vi "读取数据库.vi"(7 "condition":string, 8 "error in (no error)":errorcluster caption="错误输入（无错误）", 9 "database":string="database1.mdb", 10 "显示项":string[](array[string]), 11 "组合框":string(combo)) -> (0 "error out":errorcluster caption="错误输出", 1 "columns":string[](array[string]), 2 "data":variant[][](array[variant]), 3 "表格":string[][](table))   [LabVIEW 2016, in "数据查询.lvlib"]
uses:
  <vilib>/Utility/sysdir.llb/System Directory Type.ctl
  <vilib>/addons/database/Connection.llb/DB Tools Open Connec (String).vi
  <vilib>/addons/database/_DB Variant To Data/Database Variant To Data.xnode
  <vilib>/addons/database/NI_Database_API.lvlib
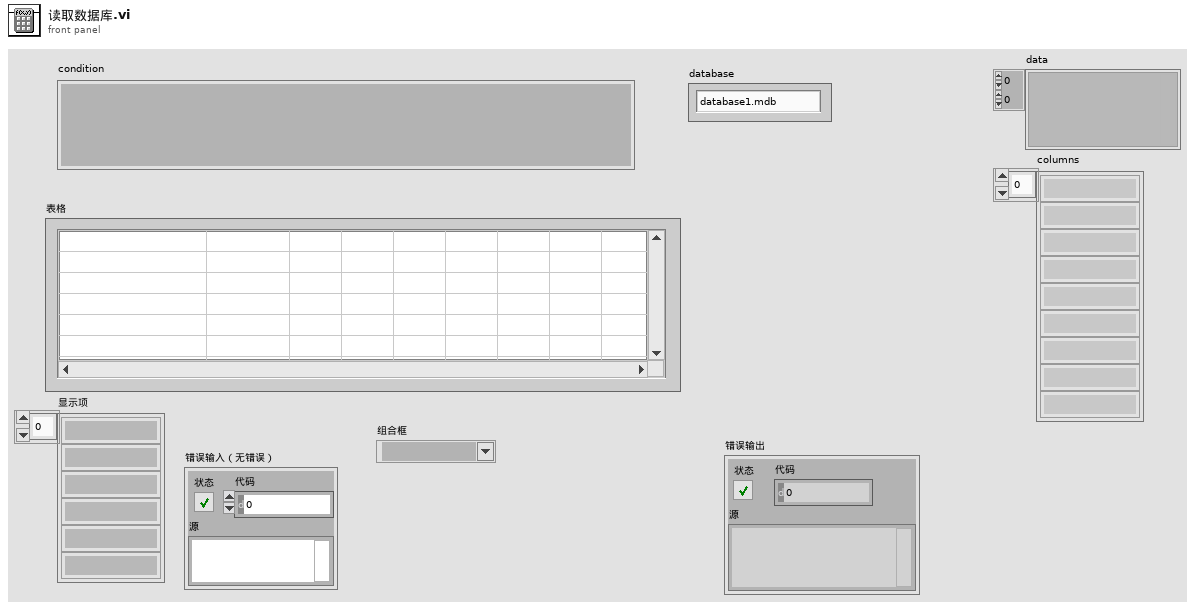
[diagram p1: front panel]
types:
  T1 = typedef "System Directory Type.ctl" = i32
  T2 = typedef "NI_Database_API.lvlib/Conn ObjectReference.ctl" = refnum<k1>
  T3 = typedef "NI_Database_API.lvlib/DB Tools DataTypes.ctl" = enum16{"String", "Long (I32)", "Single (SGL)", "Double (DBL)", "Date/Time", "Binary"}
  T4 = cluster{"name":string, "database data type":T3, "defined size":i32}[]
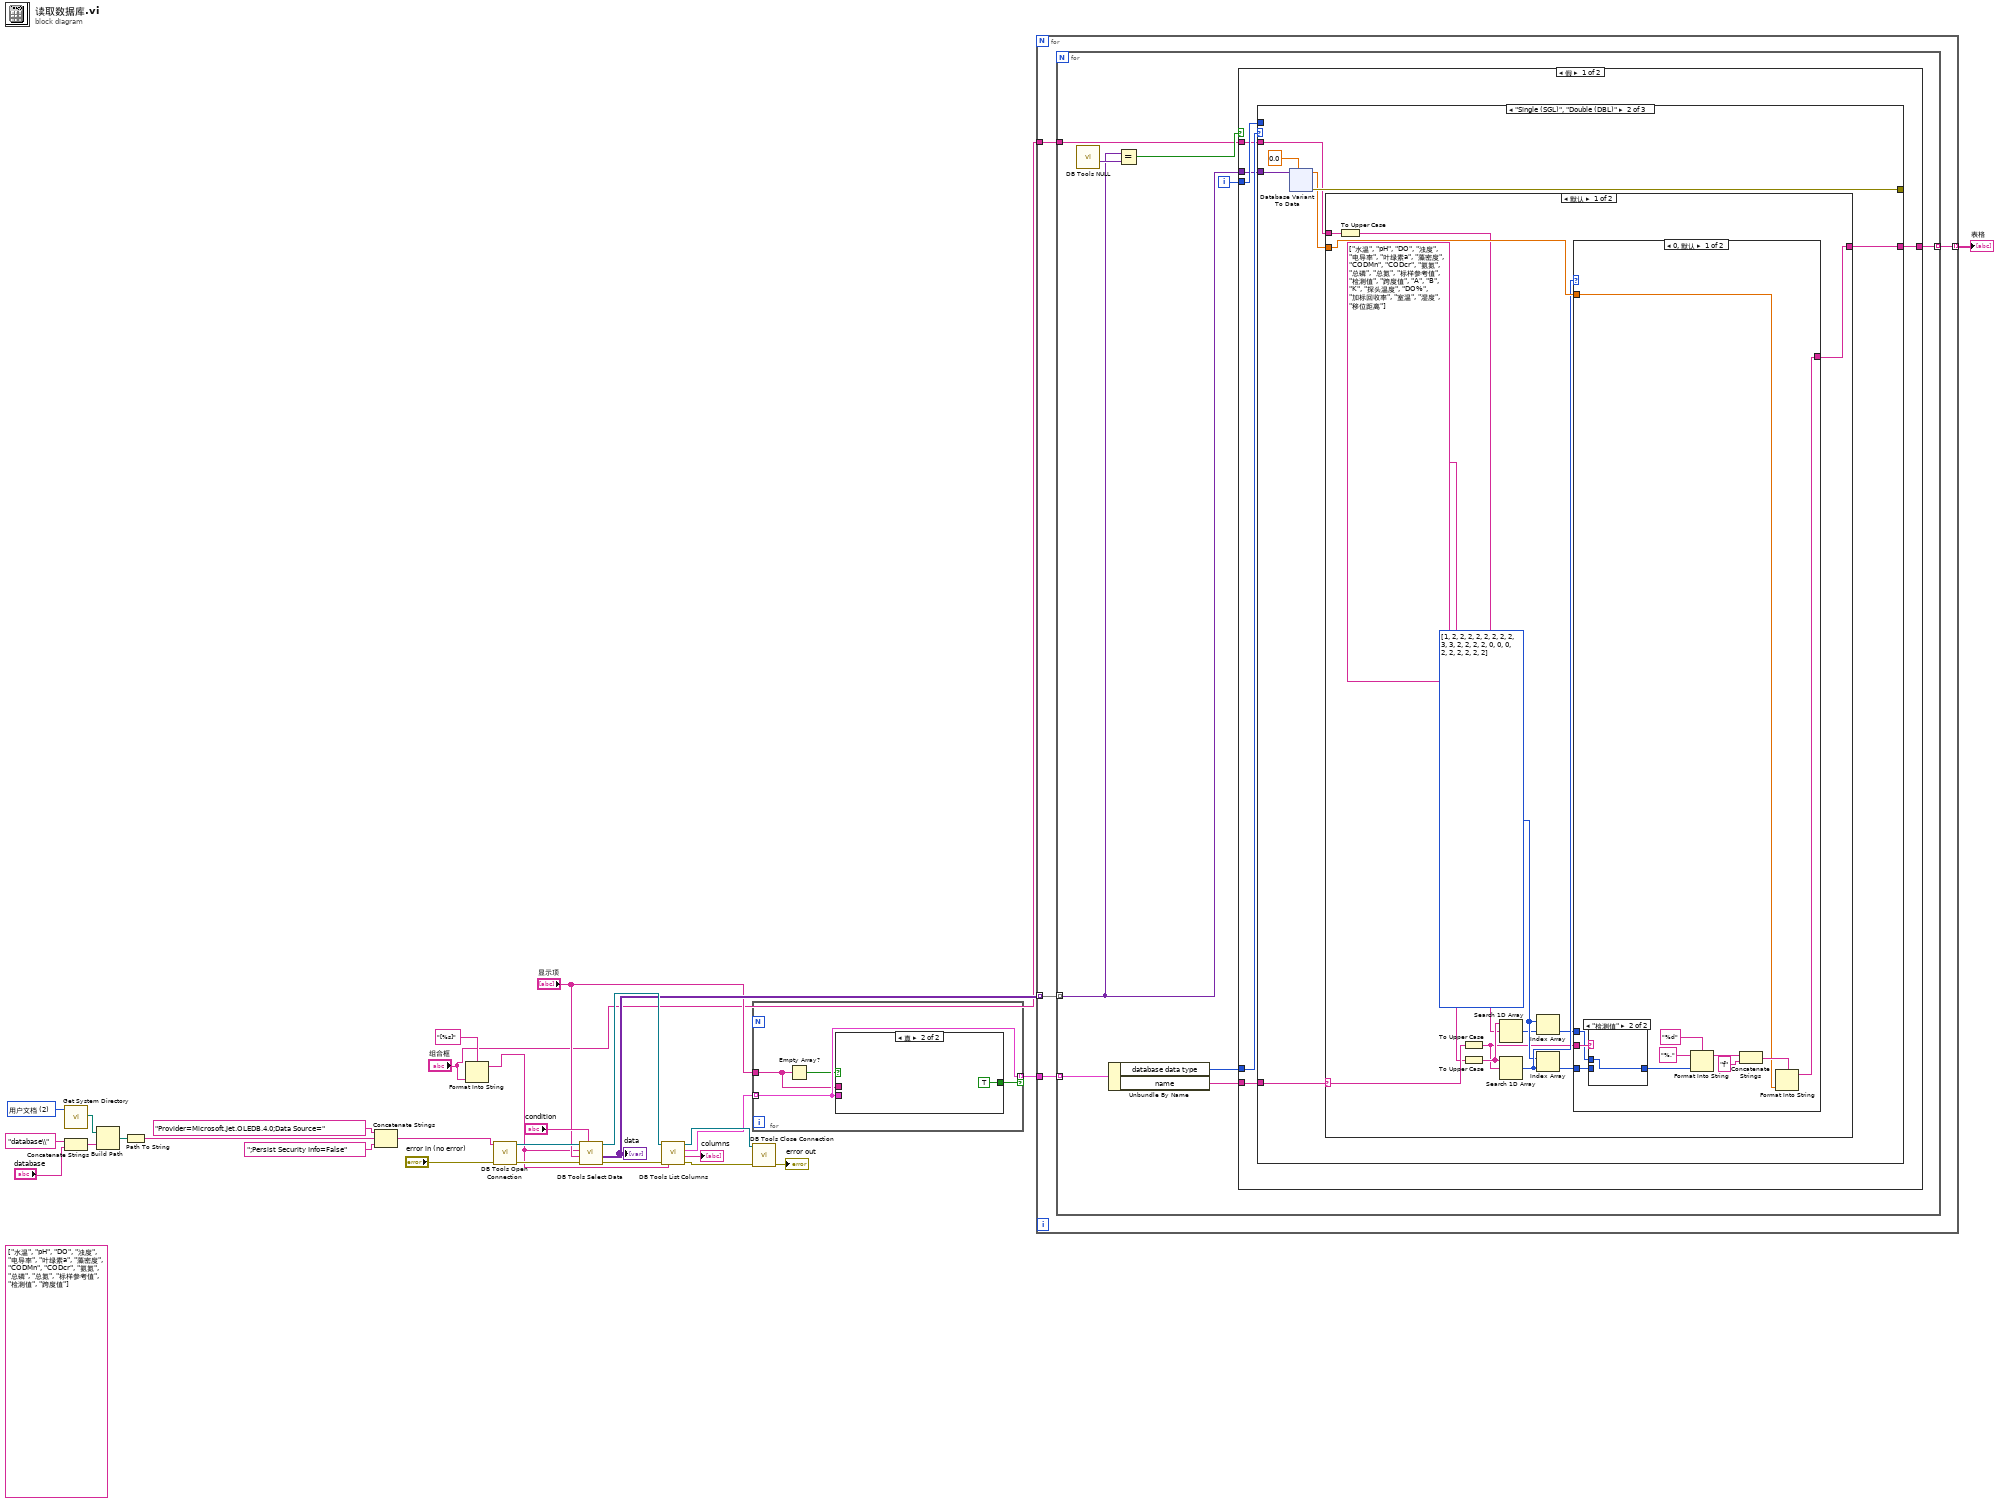
[diagram p0: block diagram]
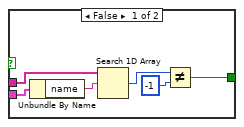
[diagram p2: hidden frame]
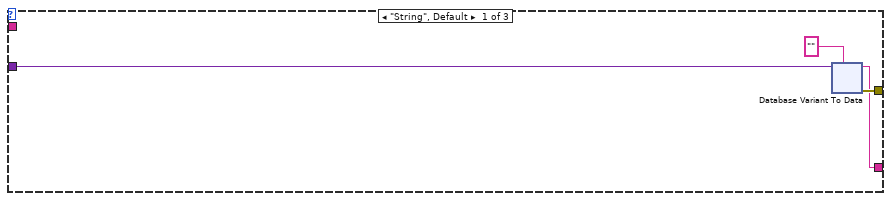
[diagram p3: hidden frame]
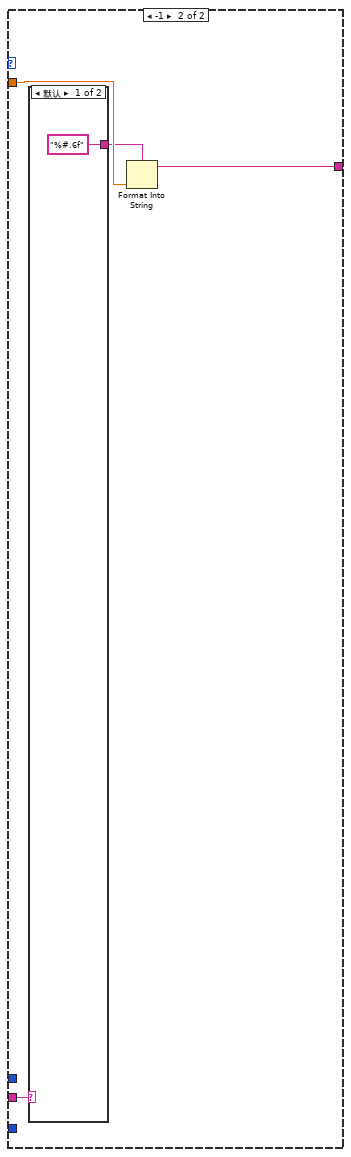
[diagram p5: hidden frame]
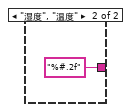
[diagram p6: hidden frame]
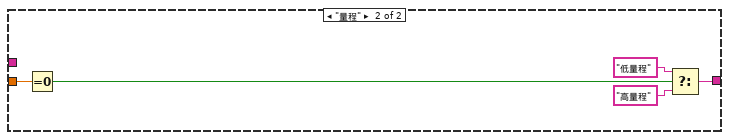
[diagram p7: hidden frame]
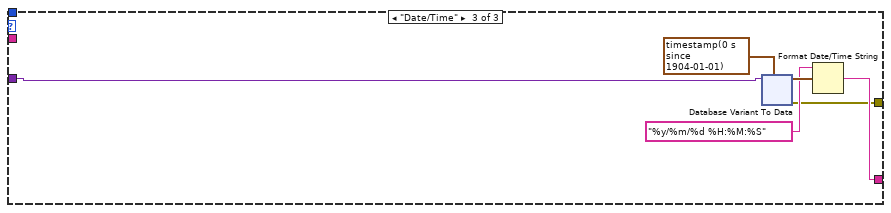
[diagram p8: hidden frame]
diagram:
  (unwired) string[] ["水温", "pH", "DO", "浊度", "电导率", "叶绿素a", "藻密度", "CODMn", "CODcr", "氨氮", "总磷", "总氮", "标样参考值", "检测值", "跨度值"]
  w15 = T1 2 items=["用户目录"=0, "用户桌面"=1, "用户文档"=2, "用户应用程序数据"=3, "用户设置"=4, "用户临时目录"=5, "公共文档"=6, "公共应用程序数据"=7, "公共设置"=8, "公共缓存"=13, "系统核心库"=9, "系统安装库"=10, "应用程序文件"=11, "启动盘根目录"=12] ("system directory type")
  n1 = call <vilib>:"Get System Directory.vi"("system directory type"=w15) -> ("system directory"=w14:path)  [unwired: 10 in]
  n2 = Concatenate Strings("database\\" ("名称或相对路径"), "database") -> (w11:string)
  n3 = Build Path(base path=w14, name or relative path=w11) -> (appended path=w16:path)
  n4 = Path To String(path=w16) -> (string=w17:string)
  n5 = Concatenate Strings("Provider=Microsoft.Jet.OLEDB.4.0;Data Source=", w17, ";Persist Security Info=False") -> (w13:string)
  n6 = Format Into String(format string="[%s]" ("格式字符串"), "组合框") -> (resulting string=w3:string)  [unwired: 2 in, 1 out]
  n7 = call-poly <vilib>:"DB Tools Open Connection.vi"("error in (no error)"="error in (no error)", "connection information"=w13) -> ("error out"=w27:errorcluster, "connection reference"=w28:T2)  [unwired: 6 in]
  n8 = call <vilib>:"DB Tools Select Data.vi"("condition"="condition", "error in (no error)"=w27, "columns"="显示项", "table"=w3, "connection reference"=w28) -> ("error out"=w26:errorcluster, "data"=w9:variant[][], "connection reference out"=w23:T2)  [unwired: 1 in]
  "data" <- w9
  n9 = call <vilib>:"DB Tools List Columns.vi"("error in (no error)"=w26, "table"=w3, "connection reference"=w23) -> ("error out"=w20:errorcluster, "columns"=→"columns":string[], "column information"=w5:T4, "connection reference out"=w21:T2)  [unwired: 1 in]
  n10 = for {
    tunnel: w5 -> [w31] mode=indexing
    tunnel: "显示项" -> [w30]
    tunnel: [w31] -> w4 mode=indexing if=w32
    n11 = Empty Array?(array=w30) -> (empty?=w29:bool)
    n12 = case shown="真" w29 {
      tunnel: [w35 TRUE] -> w32
      tunnel: w31 -> [w34 _]
      tunnel: w30 -> [w33 _]
      frame False {
        n13 = Unbundle By Name(w34) -> ("name"=w36:string)
        n14 = Search 1D Array(1D array=w33, element=w36) -> (index of element=w38:i32)  [unwired: 1 in]
        n15 = Not Equal?(x=w38, y=-1) -> (x != y?=w35:bool)
      }
      frame True {
      }
    }
  }
  n16 = call <vilib>:"DB Tools Close Connection.vi"("error in (no error)"=w20, "connection reference"=w21) -> ("error out"=→"error out":errorcluster)  [unwired: 5 in]
  n17 = for {
    tunnel: w9 -> [w43] mode=indexing
    tunnel: w4 -> [w42]
    tunnel: [w41] -> w8 mode=indexing
    tunnel: "组合框" -> [w40]
    n18 = for {
      tunnel: w43 -> [w48] mode=indexing
      tunnel: w42 -> [w52] mode=indexing
      tunnel: [w50] -> w41 mode=indexing
      tunnel: w40 -> [w46]
      i -> [w51]
      n19 = call <vilib>:"DB Tools NULL.vi"() -> ("NULL"=w49:variant)  [unwired: 10 in, 1 out]
      n20 = Unbundle By Name(w52) -> ("database data type"=w45:T3, "name"=w44:string)
      n21 = Equal?(x=w48, y=w49) -> (x = y?=w47:bool)
      n22 = case shown="假" w47 {
        tunnel: w45 -> [w58 _]
        tunnel: w51 -> [w57 _]
        tunnel: [w56 _] -> w50
        tunnel: w44 -> [w55 _]
        tunnel: w48 -> [w54 _]
        tunnel: w46 -> [w53 _]
        frame False {
          n23 = case shown="\"Single (SGL)\", \"Double (DBL)\"" w58 {
            tunnel: w54 -> [w62 w99 w176]
            tunnel: [w59 w100 w172] -> w56
            tunnel: w57 -> [_ _ _]
            tunnel: [w60 w101 w171] -> _
            tunnel: w55 -> [_ w98 _]
            tunnel: w53 -> [_ w95 _]
            frame "String", Default {
              n24 = xnode "Database Variant To Data"("database variant"=w62, "type"="") -> ("data"=w59:string, "error out"=w60:errorcluster)  [unwired: 1 in]
            }
            frame "Single (SGL)", "Double (DBL)" {
              n25 = xnode "Database Variant To Data"("database variant"=w99, "type"=0.0) -> ("data"=w96:dbl, "error out"=w101:errorcluster)  [unwired: 1 in]
              n26 = case shown="默认" w98 {
                selector: w98 -> [w112 _]
                tunnel: w96 -> [w114 w138]
                tunnel: [w113 w134] -> w100
                tunnel: w95 -> [w110 _]
                frame Default {
                  w109 = i32[] [1, 2, 2, 2, 2, 2, 2, 2, 2, 3, 3, 2, 2, 2, 2, 0, 0, 0, 2, 2, 2, 2, 2, 2]
                  n27 = To Upper Case(1:w110) -> (0:w103:string)
                  n28 = To Upper Case(1:w112) -> (0:w102:string)
                  n29 = To Upper Case(1:string[] ["水温", "pH", "DO", "浊度", "电导率", "叶绿素a", "藻密度", "CODMn", "CODcr", "氨氮", "总磷", "总氮", "标样参考值", "检测值", "跨度值", "A", "B", "K", "探头温度", "DO%", "加标回收率", "室温", "湿度", "移位距离"]) -> (0:w104:string[])
                  n30 = Search 1D Array(1D array=w104, element=w103) -> (index of element=w108:i32)  [unwired: 1 in]
                  n31 = Search 1D Array(1D array=w104, element=w102) -> (index of element=w111:i32)  [unwired: 1 in]
                  n32 = Index Array(array=w109, index=w108) -> (element=w107:i32)
                  n33 = Index Array(array=w109, index=w111) -> (element=w106:i32)
                  n34 = case shown="0, 默认" w111 {
                    tunnel: w114 -> [w119 w131]
                    tunnel: [w117 w130] -> w113
                    tunnel: w102 -> [w118 w128]
                    tunnel: w107 -> [w116 _]
                    tunnel: w106 -> [w115 _]
                    frame 0, Default {
                      n35 = case shown="\"检测值\"" w118 {
                        tunnel: [w126 w127] -> w125
                        tunnel: w116 -> [_ w127]
                        tunnel: w115 -> [w126 _]
                        frame Default {
                        }
                        frame "检测值" {
                        }
                      }
                      n36 = Format Into String(format string="%d" ("格式字符串"), initial string="%." ("初始字符串"), w125) -> (resulting string=w123:string)  [unwired: 1 in, 1 out]
                      n37 = Concatenate Strings(w123, "f" ("格式字符串")) -> (w121:string)
                      n38 = Format Into String(format string=w121, w119) -> (resulting string=w117:string)  [unwired: 2 in, 1 out]
                    }
                    frame -1 {
                      n39 = case shown="默认" w128 {
                        tunnel: ["%#.6f" ("格式字符串") "%#.2f" ("格式字符串")] -> w129
                        frame Default {
                        }
                        frame "湿度", "温度" {
                        }
                      }
                      n40 = Format Into String(format string=w129, w131) -> (resulting string=w130:string)  [unwired: 2 in, 1 out]
                    }
                  }
                }
                frame "量程" {
                  n41 = Equal To 0?(x=w138) -> (x = 0?=w137:bool)
                  n42 = Select(t="低量程" ("格式字符串"), s=w137, f="高量程" ("格式字符串")) -> (s? t:f=w134:string)
                }
              }
            }
            frame "Date/Time" {
              n43 = xnode "Database Variant To Data"("database variant"=w176, "type"=timestamp(0 s since 1904-01-01) ("当前时间")) -> ("data"=w175:timestamp, "error out"=w171:errorcluster)  [unwired: 1 in]
              n44 = Format Date/Time String(time format string (%c)="%y/%m/%d %H:%M:%S" ("时间格式字符串(%c)"), seconds (now)=w175) -> (date/time string=w172:string)  [unwired: 1 in]
            }
          }
        }
        frame True {
        }
      }
    }
  }
  "表格" <- w8
